vi "get all unexplored neighbours.vi"(2 "square (chessboard index)":T1, 3 "chessboard":T2[][](array[typedef])) -> (0 "no. of unexplored neighbours":i32, 1 "unexplored neighbours":T1[](array[typedef]))   [LabVIEW 2020, in "core.lvlib"]
uses:
  core_data/chess_square.ctl
  core_data/neighbour_square.ctl
  core_data/chessboard_index.ctl
  core.lvlib
  core_data/core_data.lvlib
panel:
  # "Development\ncontrols/indicators useful for development and testing, but which are not outputs of the VI"
  # "Input\nInputs to the VI"
  # "Output\nOutputs of the VI"
  # "Description\n\nBlank VI with error handling case. \n\nSummarize the use of this VI in this space."
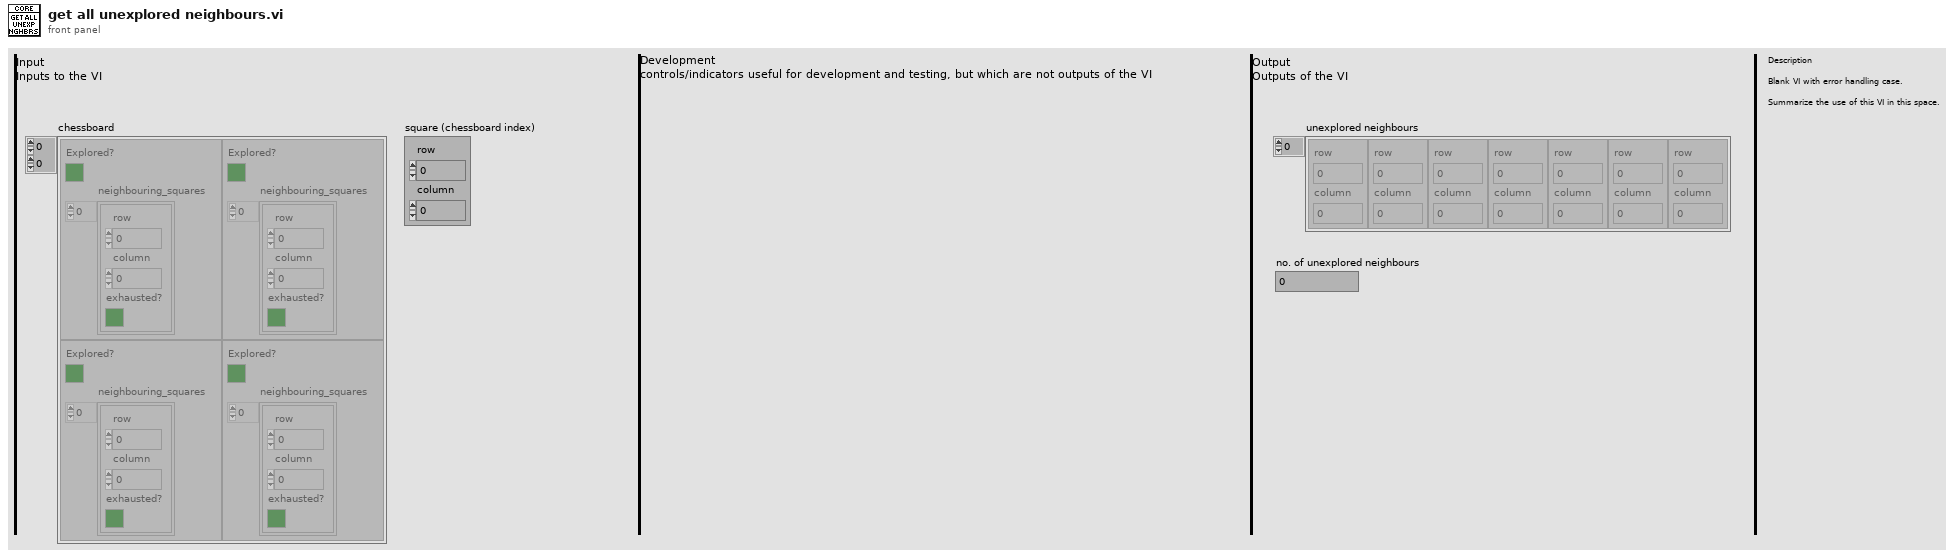
[diagram p1: front panel]
types:
  T1 = typedef "core.lvlib/core_data.lvlib/chessboard_index.ctl" = cluster{"row":u8, "column":u8}
  T2 = typedef "core.lvlib/core_data.lvlib/chess_square.ctl" = cluster{"Explored?":bool, "neighbouring_squares":T3[]}
  T3 = typedef "core.lvlib/core_data.lvlib/neighbour_square.ctl" = cluster{"row":u8, "column":u8, "exhausted?":bool}
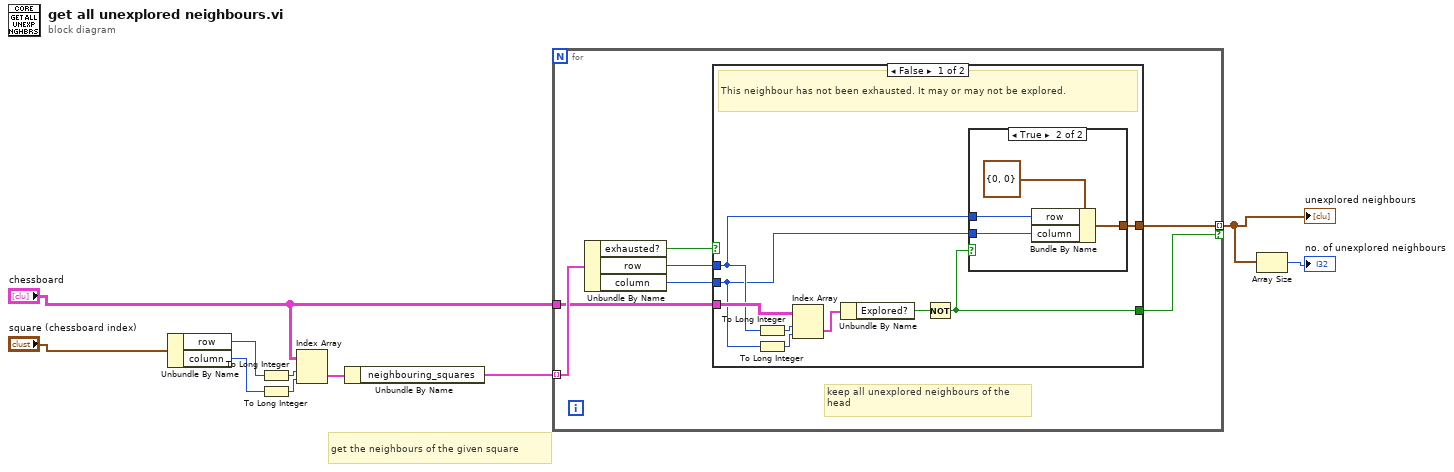
[diagram p0: block diagram]
diagram:
  # "get the neighbours of the given square"
  n1 = Unbundle By Name("square (chessboard index)") -> ("row"=w7:u8, "column"=w6:u8)
  n2 = To Long Integer(number=w7) -> (32bit integer=w5:i32)
  n3 = To Long Integer(number=w6) -> (32bit integer=w4:i32)
  n4 = Index Array(array="chessboard", index (row)=w5, index (col)=w4) -> (element=w8:T2)
  n5 = Unbundle By Name(w8) -> ("neighbouring_squares"=w9:T3[])
  n6 = for {
    tunnel: w9 -> [w16] mode=indexing
    tunnel: "chessboard" -> [w15]
    tunnel: [w11] -> w2 mode=indexing if=w12
    # "keep all unexplored neighbours of the head"
    n7 = Unbundle By Name(w16) -> ("exhausted?"=w17:bool, "row"=w14:u8, "column"=w13:u8)
    n8 = case shown="False" w17 {
      tunnel: w15 -> [w22 _]
      tunnel: w14 -> [w20 _]
      tunnel: w13 -> [w19 _]
      tunnel: [w18 _] -> w12
      tunnel: [w25 _] -> w11
      frame False {
        # "This neighbour has not been exhausted. It may or may not be explored."
        n9 = To Long Integer(number=w20) -> (32bit integer=w24:i32)
        n10 = To Long Integer(number=w19) -> (32bit integer=w23:i32)
        n11 = Index Array(array=w22, index (row)=w24, index (col)=w23) -> (element=w21:T2)
        n12 = Unbundle By Name(w21) -> ("Explored?"=w26:bool)
        n13 = Not(x=w26) -> (.not. x?=w18:bool)
        n14 = case shown="True" w18 {
          tunnel: [_ w29] -> w25
          tunnel: w20 -> [_ w28]
          tunnel: w19 -> [_ w27]
          frame False {
          }
          frame True {
            n15 = Bundle By Name(cluster=T1 {"row"=0, "column"=0} ("square_to_move_forward_to"), "row"=w28, "column"=w27) -> (w29:T1)
          }
        }
      }
      frame True {
        # "A neighbour that is exhausted is, implicitly, one that has been explored."
      }
    }
  }
  "unexplored neighbours" <- w2
  n16 = Array Size(array=w2) -> (size(s)=→"no. of unexplored neighbours":i32)
